vi "MCM3000PositionTest.vi"() -> ()   [LabVIEW 2021]
uses:
  inc/MCM3000.lvlib
panel:
  out "ZPosSlider":dbl(slide) caption="Z (mm)" min=-3.0 max=3.0 scale=-3.0..3.0
  in  "Z Stop":bool
  in  "Z Set Zero":bool
  in  "Tear Down Device and Stop Communication":bool
  out "status":i32
  in  "Move to New ZPos":bool
  in  "New ZPos (mm)":dbl
  out "Current ZPos (mm)":dbl
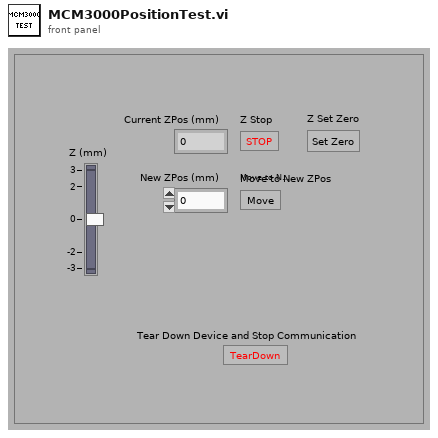
[diagram p1: front panel]
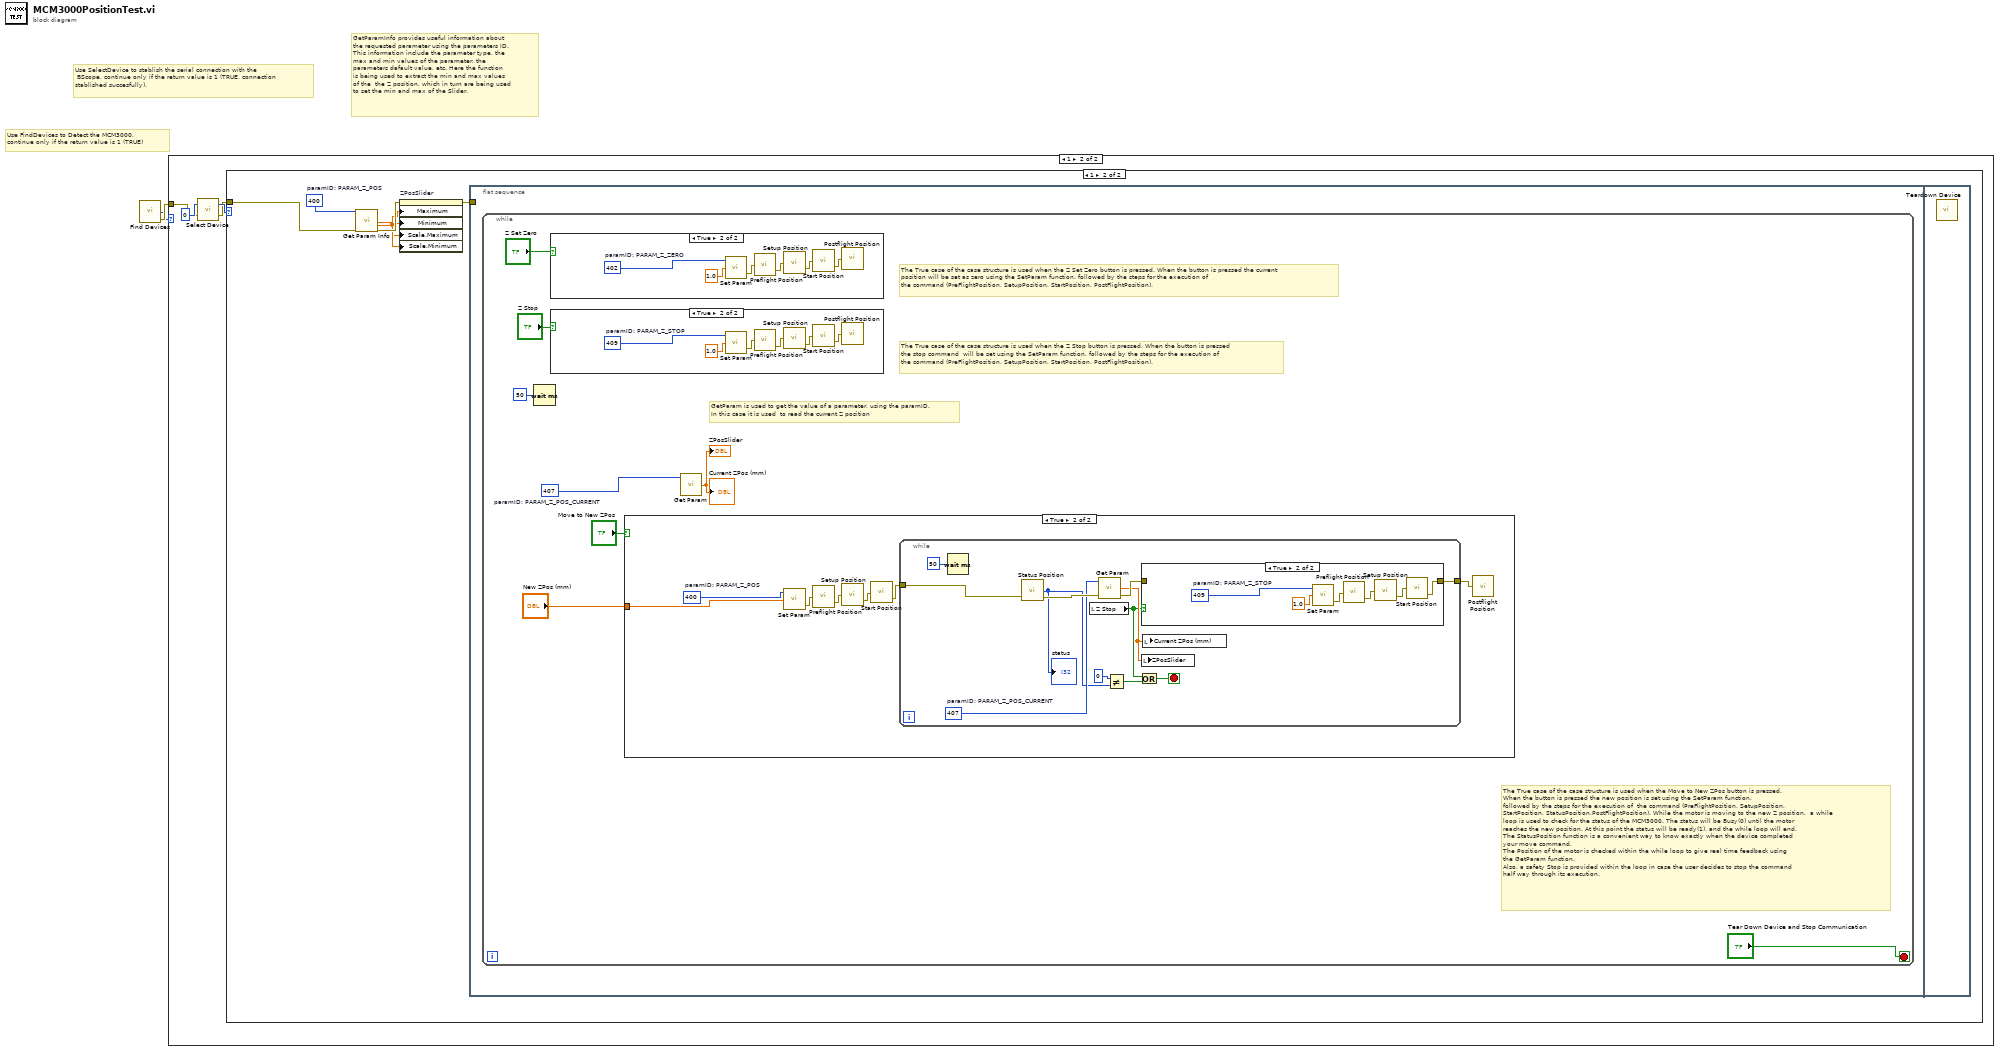
[diagram p0: block diagram]
diagram:
  # "GetParamInfo provides useful information about \nthe requested parameter using the parameters ID.\nThis information include the parameter type, the \nmax and min values of the parameter, the \nparameters dafault value, etc. Here the function \nis being used to extract the min and max values \nof the  the Z position, which in turn are being used\nto set the min and max of the Slider."
  # "Use SelectDevice to stablish the serial connection with the\n BScope, continue only if the return value is 1 (TRUE, connection\nstablished succesfully)."
  # "Use FindDevices to Detect the MCM3000, \ncontinue only if the return value is 1 (TRUE)"
  n1 = call "Find Devices.vi"() -> ("function return"=w1:i32, "error out"=w2:errorcluster)  [unwired: 2 in, 1 out]
  n2 = case shown="1" w1 {
    tunnel: w2 -> [_ w5]
    frame 0, Default {
    }
    frame 1 {
      n3 = call "Select Device.vi"("error in (no error)"=w5, "Device"=0) -> ("error out"=w3:errorcluster, "function return"=w4:i32)
      n4 = case shown="1" w4 {
        tunnel: w3 -> [_ w12]
        frame 0, Default {
        }
        frame 1 {
          w7 = 400  # paramID: PARAM_Z_POS
          n5 = call "Get Param Info.vi"("paramID"=w7, "error in (no error)"=w12) -> ("paramMin out"=w9:dbl, "paramMax out"=w8:dbl, "error out"=w10:errorcluster)  [unwired: 18 in, 5 out]
          n6 = property on="ZPosSlider" class="Slide (strict)"(error in=w10, "Maximum"=w8, "Minimum"=w9, "Scale.Maximum"=w8, "Scale.Minimum"=w9) -> (error out=w11:errorcluster)  [unwired: 1 in, 1 out]
          n7 = flat-sequence {
            tunnel: w11 -> [_]
            frame #0 {
              n8 = while {
                stop <- "Tear Down Device and Stop Communication" stop-if-true
                w18 = 407  # paramID: PARAM_Z_POS_CURRENT
                # "The True case of the case structure is used when the Move to New ZPos button is pressed. \nWhen the button is pressed the new position is set using the SetParam function, \nfollowed by the steps for the execution of  the command (PreFlightPosition, SetupPosition, \nStartPosition, StatusPosition,PostFlightPosition). While the motor is moving to the new Z position,  a while \nloop is used to check for the status of the MCM3000. The status will be Busy(0) until the motor\nreaches the new position. At this point the status will be ready(1), and the while loop will end.\nThe StatusPosition function is a convenient way to know exactly when the device completed\nyour move command.\nThe Position of the motor is checked within the while loop to give real time feedback using \nthe GetParam function.\nAlso, a safety Stop is provided within the loop in case the user decides to stop the command \nhalf way through its execution."
                # "The True case of the case structure is used when the Z Stop button is pressed. When the button is pressed\nthe stop command  will be set using the SetParam function, followed by the steps for the execution of \nthe command (PreFlightPosition, SetupPosition, StartPosition, PostFlightPosition)."
                # "GetParam is used to get the value of a parameter, using the paramID.\nIn this case it is used  to read the current Z position"
                # "The True case of the case structure is used when the Z Set Zero button is pressed. When the button is pressed the current\nposition will be set as zero using the SetParam function, followed by the steps for the execution of \nthe command (PreFlightPosition, SetupPosition, StartPosition, PostFlightPosition)."
                n9 = Wait (ms)(milliseconds to wait=u32 50) -> ()  [unwired: 1 out]
                n10 = case shown="True" "Z Set Zero" {
                  frame False {
                  }
                  frame True {
                    w31 = 402  # paramID: PARAM_Z_ZERO
                    n11 = call "Set Param.vi"("param"=1.0, "paramID"=w31) -> ("error out"=w30:errorcluster)  [unwired: 1 in, 1 out]
                    n12 = call "Preflight Position.vi"("error in (no error)"=w30) -> ("error out"=w29:errorcluster)  [unwired: 1 out]
                    n13 = call "Setup Position.vi"("error in (no error)"=w29) -> ("error out"=w28:errorcluster)  [unwired: 1 out]
                    n14 = call "Start Position.vi"("error in (no error)"=w28) -> ("error out"=w27:errorcluster)  [unwired: 1 out]
                    n15 = call "Postflight Position.vi"("error in (no error)"=w27) -> ()  [unwired: 2 out]
                  }
                }
                n16 = case shown="True" "Z Stop" {
                  frame False {
                  }
                  frame True {
                    w25 = 409  # paramID: PARAM_Z_STOP
                    n17 = call "Set Param.vi"("param"=1.0, "paramID"=w25) -> ("error out"=w24:errorcluster)  [unwired: 1 in, 1 out]
                    n18 = call "Preflight Position.vi"("error in (no error)"=w24) -> ("error out"=w23:errorcluster)  [unwired: 1 out]
                    n19 = call "Setup Position.vi"("error in (no error)"=w23) -> ("error out"=w22:errorcluster)  [unwired: 1 out]
                    n20 = call "Start Position.vi"("error in (no error)"=w22) -> ("error out"=w21:errorcluster)  [unwired: 1 out]
                    n21 = call "Postflight Position.vi"("error in (no error)"=w21) -> ()  [unwired: 2 out]
                  }
                }
                n22 = case shown="True" "Move to New ZPos" {
                  tunnel: "New ZPos (mm)" -> [_ w35]
                  frame False {
                  }
                  frame True {
                    w37 = 400  # paramID: PARAM_Z_POS
                    n23 = call "Set Param.vi"("param"=w35, "paramID"=w37) -> ("error out"=w36:errorcluster)  [unwired: 1 in, 1 out]
                    n24 = call "Preflight Position.vi"("error in (no error)"=w36) -> ("error out"=w39:errorcluster)  [unwired: 1 out]
                    n25 = call "Setup Position.vi"("error in (no error)"=w39) -> ("error out"=w38:errorcluster)  [unwired: 1 out]
                    n26 = call "Start Position.vi"("error in (no error)"=w38) -> ("error out"=w34:errorcluster)  [unwired: 1 out]
                    n27 = while {
                      tunnel: w34 -> [w47]
                      tunnel: [w45] -> w33
                      stop <- w41 stop-if-true
                      w48 = 407  # paramID: PARAM_Z_POS_CURRENT
                      n28 = Wait (ms)(milliseconds to wait=u32 50) -> ()  [unwired: 1 out]
                      n29 = call "Status Position.vi"("error in (no error)"=w47) -> ("function return"=w43:i32, "error out"=w49:errorcluster)  [unwired: 1 in, 1 out]
                      "status" <- w43
                      n30 = local read "Z Stop"() -> (w40:bool)
                      n31 = call "Get Param.vi"("error in (no error)"=w49, "paramID"=w48) -> ("error out"=w46:errorcluster, "param out"=w44:dbl)  [unwired: 1 in, 1 out]
                      n32 = Not Equal?(x=0, y=w43) -> (x != y?=w42:bool)
                      n33 = Or(x=w40, y=w42) -> (x .or. y?=w41:bool)
                      n34 = case shown="True" w40 {
                        tunnel: w46 -> [w52 _]
                        tunnel: [w52 w53] -> w45
                        frame False {
                        }
                        frame True {
                          w57 = 409  # paramID: PARAM_Z_STOP
                          n35 = call "Set Param.vi"("param"=1.0, "paramID"=w57) -> ("error out"=w56:errorcluster)  [unwired: 1 in, 1 out]
                          n36 = call "Preflight Position.vi"("error in (no error)"=w56) -> ("error out"=w55:errorcluster)  [unwired: 1 out]
                          n37 = call "Setup Position.vi"("error in (no error)"=w55) -> ("error out"=w54:errorcluster)  [unwired: 1 out]
                          n38 = call "Start Position.vi"("error in (no error)"=w54) -> ("error out"=w53:errorcluster)  [unwired: 1 out]
                        }
                      }
                      n39 = local write "ZPosSlider"(w44) -> ()
                      n40 = local write "Current ZPos (mm)"(w44) -> ()
                    }
                    n41 = call "Postflight Position.vi"("error in (no error)"=w33) -> ()  [unwired: 2 out]
                  }
                }
                n42 = call "Get Param.vi"("paramID"=w18) -> ("param out"=→"Current ZPos (mm)" →"ZPosSlider":dbl)  [unwired: 2 in, 2 out]
              }
            }
            frame #1 {
              n43 = call "Teardown Device.vi"() -> ()  [unwired: 1 in, 2 out]
            }
          }
        }
      }
    }
  }
